vi "变更显示.vi"(8 "error in":errorcluster caption="错误输入（无错误）", 11 "仓库路径":path=path "E:/学习文件/Git插件/test") -> (0 "error out":errorcluster caption="错误输出", 1 "standard error":string caption="标准错误", 2 "变更项":string[](array[string]), 3 "仓库路径":path=path "E:/学习文件/Git插件/test")   [LabVIEW 2018]
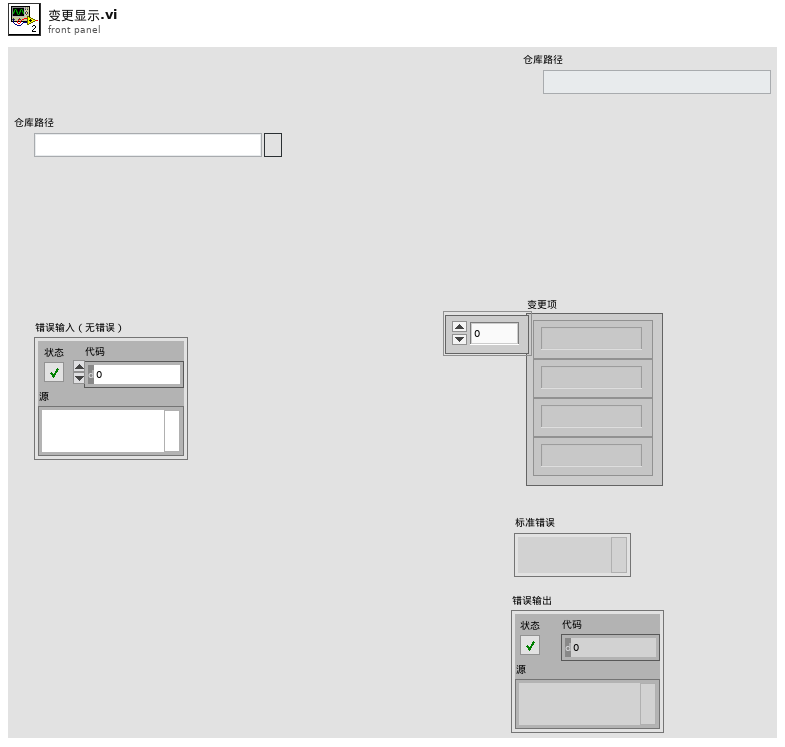
[diagram p1: front panel]
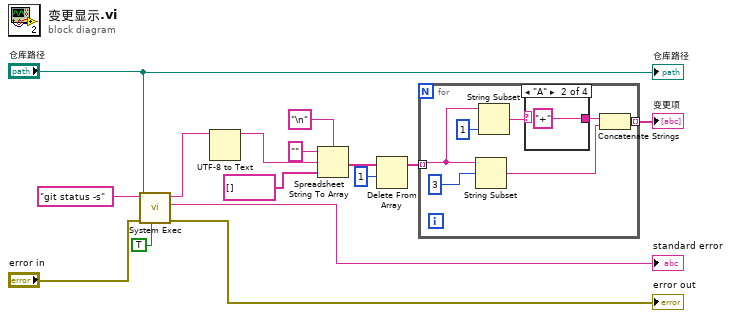
[diagram p0: block diagram]
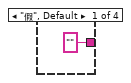
[diagram p2: hidden frame]
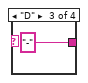
[diagram p3: hidden frame]
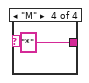
[diagram p4: hidden frame]
diagram:
  n1 = call <vilib>:"System Exec.vi"("run minimized? (F)"=TRUE, "error in (no error)"="error in", "working directory"="仓库路径", "command line"="git status -s") -> ("error out"=→"error out":errorcluster, "standard error"=→"standard error":string, "standard output"=w13:string)  [unwired: 4 in, 1 out]
  n2 = UTF-8 to Text ("UTF-8至文本转换")(11:w13) -> (3:w9:string)  [unwired: 2 in, 1 out]
  n3 = Spreadsheet String To Array(delimiter (Tab)="\n" ("分隔符(Tab)"), format string="" ("格式字符串"), spreadsheet string=w9, array type (2D Dbl)=string[] []) -> (array=w4:string[])
  n4 = Delete From Array(array=w4, length=1 ("长度")) -> (array with subset deleted=w2:string[])  [unwired: 1 in, 1 out]
  n5 = for {
    tunnel: w2 -> [w21] mode=indexing
    tunnel: [w16] -> w1 mode=indexing
    n6 = String Subset(string=w21, offset (0)=3 ("偏移量(0)")) -> (substring=w17:string)  [unwired: 1 in]
    n7 = String Subset(string=w21, length (rest)=1 ("长度（剩余）")) -> (substring=w19:string)  [unwired: 1 in]
    n8 = case shown="\"A\"" w19 {
      tunnel: ["" "+" "-" "*"] -> w18
      frame "假", Default {
      }
      frame "A" {
      }
      frame "D" {
      }
      frame "M" {
      }
    }
    n9 = Concatenate Strings(w18, w17) -> (w16:string)
  }
  "变更项" <- w1
  "仓库路径" <- "仓库路径"
